vi "enum_saved_default.vi"(10 "mode":enum16{"Idle", "Run"}(ring)=enum."Run") -> (2 "result":enum16{"Idle", "Run"}(ring))   [LabVIEW 2020]
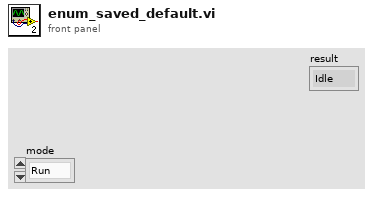
[diagram p1: front panel]
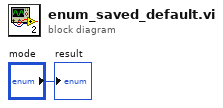
[diagram p0: block diagram]
diagram:
  "result" <- "mode"
